vi "7) Case Structure.vi"() -> ()   [LabVIEW 2018]
panel:
  in  "Numeric":dbl
  in  "Temperature (F)":dbl(slide) scale=0.0..100.0
  out "Temperature (C)":dbl(slide) scale=0.0..100.0
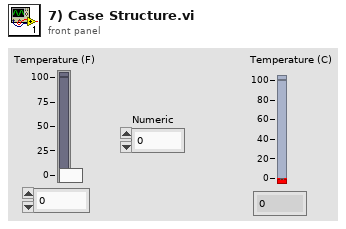
[diagram p1: front panel]
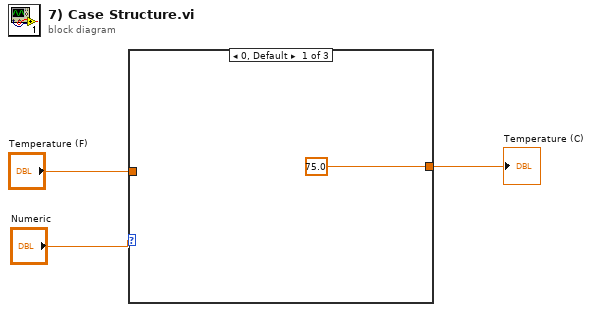
[diagram p0: block diagram]
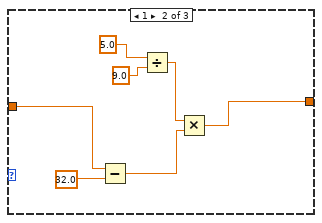
[diagram p2: hidden frame]
diagram:
  n1 = case shown="0, Default" "Numeric" {
    tunnel: [75.0 ("Temperature (F)") w9 w12] -> w3
    tunnel: "Temperature (F)" -> [_ w7 w12]
    frame 0, Default {
    }
    frame 1 {
      n2 = Subtract(x=w7, y=32.0 ("x-y")) -> (x-y=w10:dbl)
      n3 = Divide(x=5.0 ("x/y"), y=9.0) -> (x/y=w11:dbl)
      n4 = Multiply(x=w11, y=w10) -> (x*y=w9:dbl)
    }
    frame 2 {
    }
  }
  "Temperature (C)" <- w3
